vi "stopUI.vi"(8 "error in (no error)":errorcluster, 10 "UI VI*":refnum<vi>, 11 "xceDataNode in":refnum<class "xceDataNode.lvclass">) -> (0 "error out":errorcluster, 3 "xceDataNode out":refnum<class "xceDataNode.lvclass">)   [LabVIEW 2013, in "xceDataNode.lvclass"]
doc: "Stops the user interface VI for this xceDataNode. This is the end to unloading the UI VI into the xceSubpanel class. Also this VI is dynamic dispatch because it is just the suggested way to stop a dynamic VI. This has been created with the idea that your classes UI VI will be created from the DataNodeUI.vit template."
uses:
  xceDataNode.lvclass
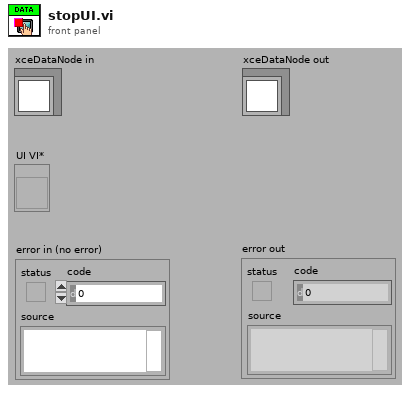
[diagram p1: front panel]
types:
  T1 = enum32{"Bad", "Idle", "Run top level", "Running"}
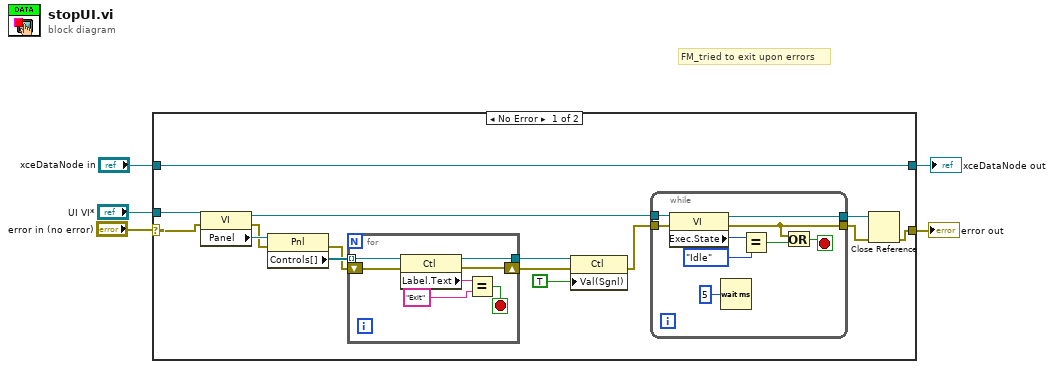
[diagram p0: block diagram]
diagram:
  # "FM_tried to exit upon errors"
  n1 = case shown="No Error" "error in (no error)" {
    selector: "error in (no error)" -> [w18 w38]
    tunnel: "xceDataNode in" -> [w20 w37]
    tunnel: "UI VI*" -> [w19 _]
    tunnel: [w6 w38] -> w2
    tunnel: [w20 w37] -> w1
    frame No Error {
      n2 = property class="VI"(reference=w19, error in=w18) -> (reference out=w10:refnum<vi>, error out=w16:errorcluster, "Panel"=w17:refnum<vi>)
      n3 = property class="Pnl"(reference=w17, error in=w16) -> (error out=w14:errorcluster, "Controls[]"=w15:refnum<vi>[])  [unwired: 1 out]
      n4 = for {
        tunnel: w15 -> [w36] mode=indexing
        shift-right: [w34] -> w12
        shift-left: w14 -> [w35]
        tunnel: [w30] -> w13
        stop <- w31 stop-if-true
        n5 = property class="Ctl"(reference=w36, error in=w35) -> (reference out=w30:refnum<vi>, error out=w34:errorcluster, "Label.Text"=w33:string)
        n6 = Equal?(x=w33, y="Exit" ("Label.Text")) -> (x = y?=w31:bool)
      }
      n7 = property class="Ctl"(reference=w13, error in=w12, "Val(Sgnl)"=TRUE) -> (error out=w7:errorcluster)  [unwired: 1 out]
      n8 = while {
        tunnel: w10 -> [w29]
        tunnel: [w26] -> w9
        tunnel: [w23] -> w8
        tunnel: w7 -> [w25]
        stop <- w21 stop-if-true
        n9 = property class="VI"(reference=w29, error in=w25) -> (reference out=w26:refnum<vi>, error out=w23:errorcluster, "Exec.State"=w28:T1)
        n10 = Wait (ms)(milliseconds to wait=u32 5) -> ()  [unwired: 1 out]
        n11 = Equal?(x=w28, y=T1."Idle") -> (x = y?=w22:bool)
        n12 = Or(x=w23, y=w22) -> (x .or. y?=w21:bool)
      }
      n13 = Close Reference(reference=w9, error in (no error)=w8) -> (error out=w6:errorcluster)
    }
    frame Error {
    }
  }
  "xceDataNode out" <- w1
  "error out" <- w2
